vi "ReadFileSettingControl.vi"(8 "error in":errorcluster, 10 "ThisVI_In":refnum<vi>, 11 "Path to was selected by user":path caption="selected path") -> (2 "ThisVI_Out":refnum<vi>)   [LabVIEW 2013]
uses:
  <vilib>/regexp/Match Regular Expression.xnode
panel:
  out "error out":errorcluster
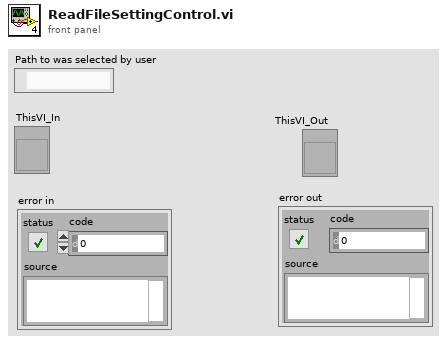
[diagram p1: front panel]
types:
  T1 = enum16{"open", "replace", "create", "open or create", "replace or create", "replace or create with confirmation"}
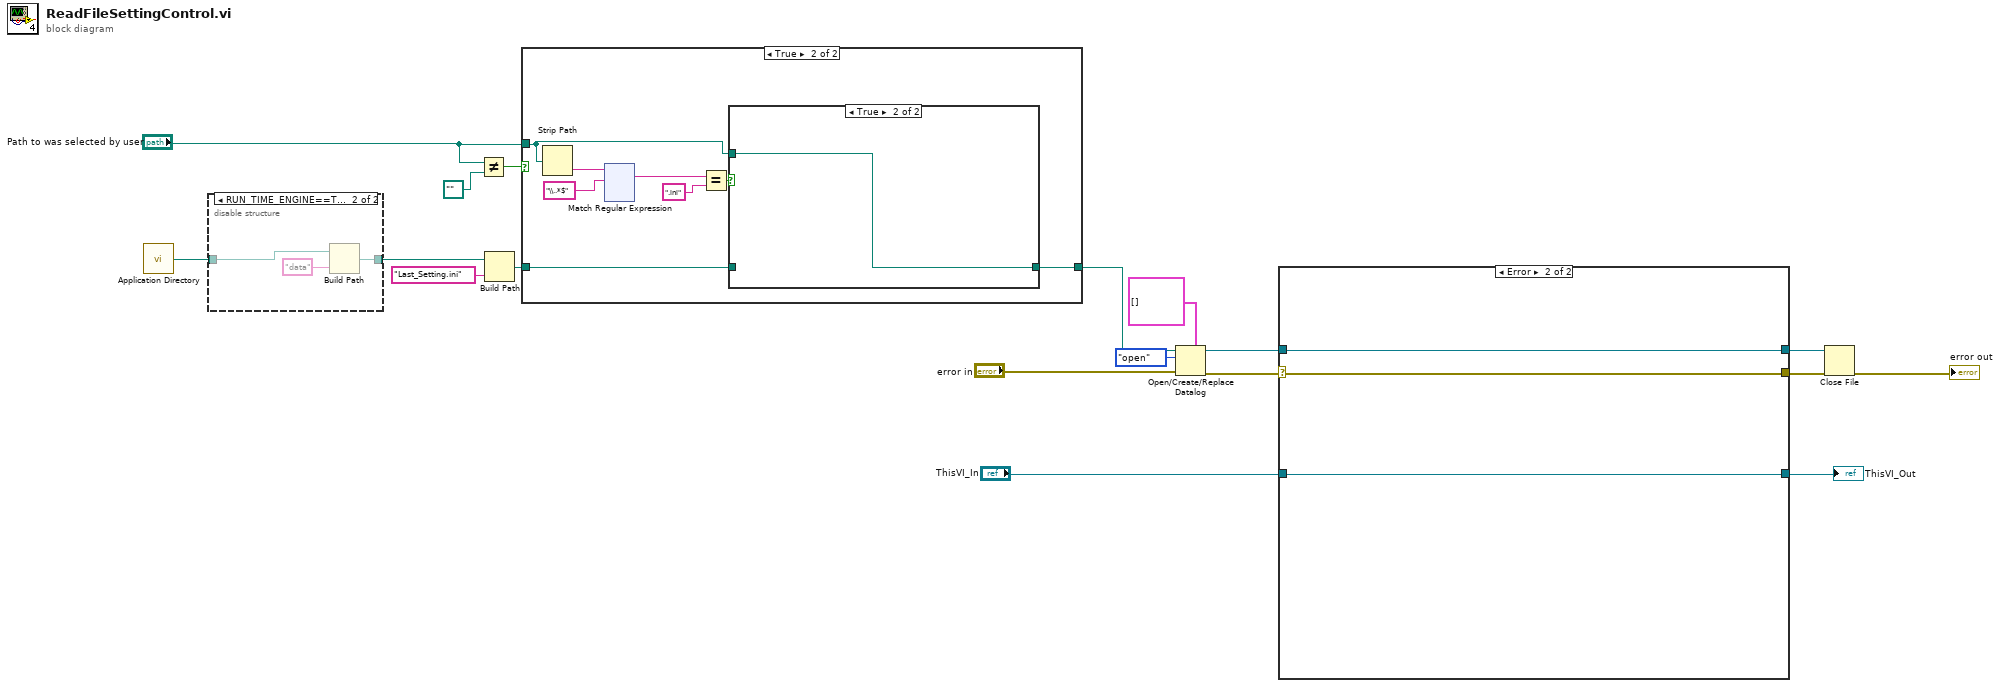
[diagram p0: block diagram]
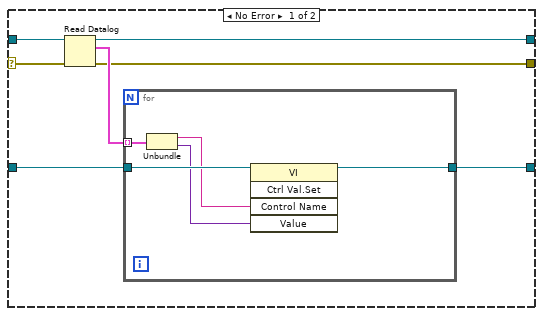
[diagram p2: hidden frame]
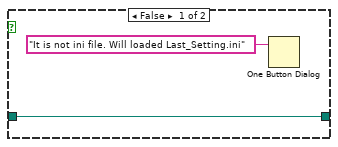
[diagram p5: hidden frame]
diagram:
  n1 = call <vilib>:"Application Directory.vi"() -> ("Application Directory"=w14:path)
  n2 = disable-structure shown="RUN_TIME_ENGINE==True" {
    disable-tunnel: w14 -> [w19 w22]
    disable-tunnel: [w19 w20] -> w15
    frame condition #0 (active) {
    }
    frame condition #1 {
      n3 = Build Path(base path=w22, name or relative path="data") -> (appended path=w20:path)
    }
  }
  n4 = Not Equal?(x="Path to was selected by user", y=path "" ("Path to folder was selected by user")) -> (x != y?=w16:bool)
  n5 = Build Path(base path=w15, name or relative path="Last_Setting.ini") -> (appended path=w12:path)
  n6 = case shown="True" w16 {
    tunnel: "Path to was selected by user" -> [_ w24]
    tunnel: w12 -> [w23 w26]
    tunnel: [w23 w25] -> w11
    frame False {
    }
    frame True {
      n7 = Strip Path(path=w24) -> (name=w31:string)  [unwired: 1 out]
      n8 = xnode "Match Regular Expression"("input string"=w31, "regular expression"="\\..*$") -> ("whole match"=w28:string)  [unwired: 4 in, 4 out]
      n9 = Equal?(x=w28, y=".ini" ("whole match")) -> (x = y?=w27:bool)
      n10 = case shown="True" w27 {
        tunnel: w24 -> [_ w34]
        tunnel: w26 -> [w33 _]
        tunnel: [w33 w34] -> w25
        frame False {
          n11 = One Button Dialog(message="It is not ini file. Will loaded Last_Setting.ini") -> ()  [unwired: 1 in, 1 out]
        }
        frame True {
        }
      }
    }
  }
  n12 = Open/Create/Replace Datalog(5:cluster{"Name":string, "Variant Data":variant}[] [] ("Control Value:Get All"), 8:"error in", 10:T1."open" ("operation (0:open)"), 11:w11) -> (0:w4:errorcluster, 3:w6:refnum<k1>)  [unwired: 2 in, 1 out]
  n13 = case shown="Error" w4 {
    selector: w4 -> [w151 w163]
    tunnel: "ThisVI_In" -> [w155 w162]
    tunnel: [w154 w162] -> w8
    tunnel: [w149 w163] -> w3
    tunnel: w6 -> [w153 w161]
    tunnel: [w150 w161] -> w1
    frame No Error {
      n14 = Read Datalog(4:w151, 7:w153) -> (0:w149:errorcluster, 2:w152:cluster{"Name":string, "Variant Data":variant}[], 3:w150:refnum<k1>)  [unwired: 1 in]
      n15 = for {
        tunnel: w152 -> [w160] mode=indexing
        tunnel: w155 -> [w159]
        tunnel: [w156] -> w154
        n16 = Unbundle(w160) -> ("Name"=w158:string, "Variant Data"=w157:variant)
        n17 = invoke class="VI" method="Ctrl Val.Set"(reference=w159, "Control Name"=w158, "Value"=w157) -> (reference out=w156:refnum<vi>)  [unwired: 2 in, 4 out]
      }
    }
    frame Error {
    }
  }
  "ThisVI_Out" <- w8
  n18 = Close File(refnum=w1, error in=w3) -> (error out=→"error out":errorcluster)  [unwired: 1 out]
